vi "Pump Message Loop.vi"(7 "Manual Pump Select":enum32{"In", "Out"}(radio), 8 "error in (no error)":errorcluster) -> (0 "error out":errorcluster)   [LabVIEW 2020, in "Pump.lvlib"]
doc: "Message loop for handling messages pertaining to the acquisition of data from the hardware."
uses:
  Pump.lvlib
  support/PCT FGV CMD.ctl
  Acquisition State.ctl
  Pump Hardware Configuration.ctl
  support/Message Queue/Message Cluster.ctl
  support/Message Queue/Enqueue Message (Single).vi
  <vilib>/Utility/error.llb/Error Cluster From Error Code.vi
  <vilib>/ErrorRing/Error Ring.xnode
  support/Message Queue/Message Queue.lvlib
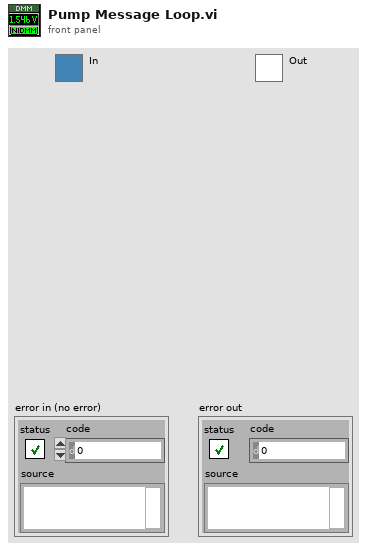
[diagram p1: front panel]
types:
  T1 = typedef "PCT FGV CMD.ctl" = enum16{"INIT", "GET", "SET"}
  T2 = typedef "PCT Data REFs.ctl" = cluster{"PLC AI Notifier":refnum<notifier>, "PS Data Queue":refnum<queue>, "BTN Queue":refnum<queue>, "PLC DI notifier":refnum<notifier>, "Timer notifier":refnum<notifier>, "DMM PS":refnum<notifier>, "DMM Gages":refnum<notifier>, "XYZ notifier":refnum<notifier>, "Test Notifier":refnum<notifier>, "Scanner notifier":refnum<notifier>, "OPC Notifier":refnum<notifier>, "HIDEN queue":refnum<queue>}
  T3 = typedef "Message Queue.lvlib/All Message Queues.ctl" = cluster{"UI":refnum<queue>, "Logging":refnum<queue>, "LOG":refnum<queue>, "ALARM":refnum<queue>, "Test":refnum<queue>, "Answer":refnum<queue>, "PLC":refnum<queue>, "DB":refnum<queue>, "Report":refnum<queue>, "OPC":refnum<queue>, "Procedure":refnum<queue>, "PalmSens":refnum<queue>, "SYS 7000 Reader":refnum<queue>, "SWITCH":refnum<queue>, "MOTOR":refnum<queue>, "MOTION":refnum<queue>, "HIDEN":refnum<queue>, "VALVE":refnum<queue>, "MFC":refnum<queue>, "PUMP IN":refnum<queue>, "PUMP OUT":refnum<queue>}
  T4 = typedef "Pump.lvlib/Pump Hardware Configuration.ctl" = cluster{"Pump  name":refnum<visa-resource-name>[], "Writer Queue":refnum<queue>, "Pump Info":cluster{"Pump Type":string, "Speed":i32, "Direction":u16, "Running":bool}, "Current Pump Name":refnum<visa-resource-name>, "Wait":dbl, "Next Step":string, "Reset":bool}
  T5 = cluster{"Type CMD":string, "Mode CMD":string, "Main CMD":string}
  T6 = typedef "Pump.lvlib/Acquisition State.ctl" = enum16{"Idle", "Initialized"}
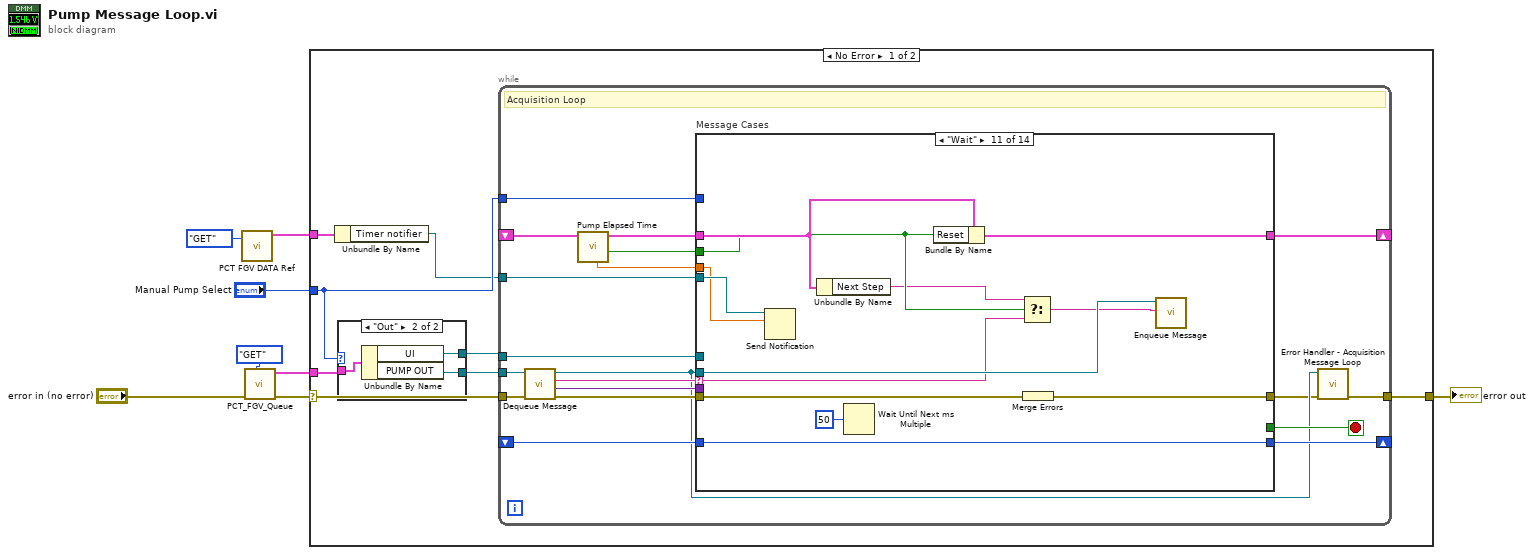
[diagram p0: block diagram]
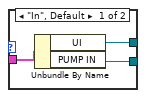
[diagram p2: hidden frame]
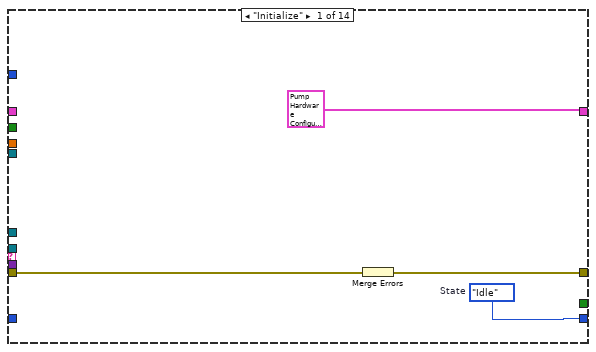
[diagram p3: hidden frame]
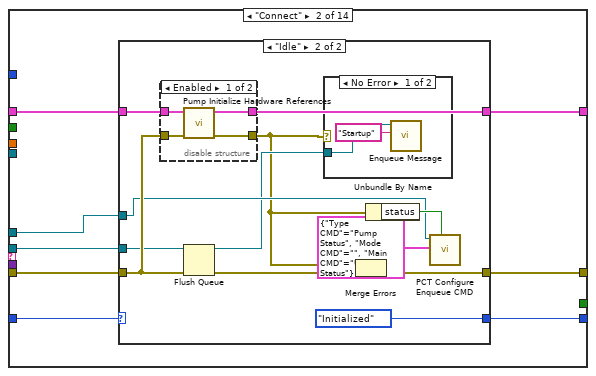
[diagram p4: hidden frame]
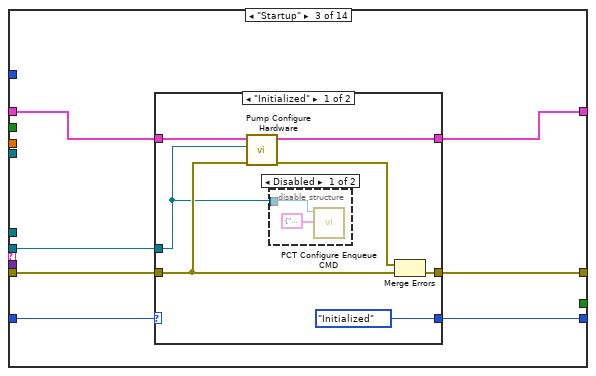
[diagram p8: hidden frame]
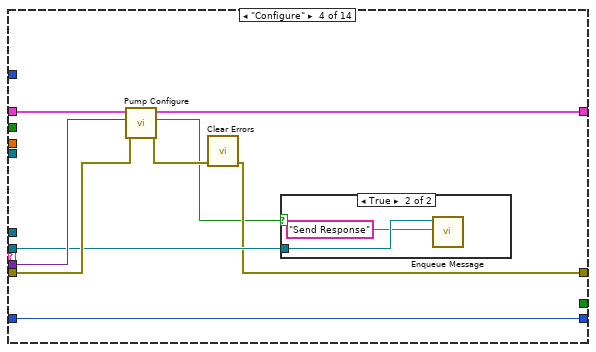
[diagram p11: hidden frame]
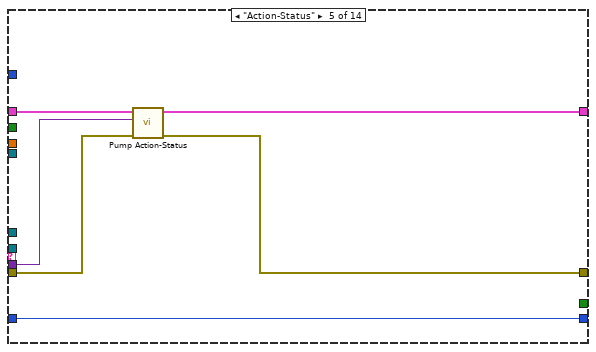
[diagram p13: hidden frame]
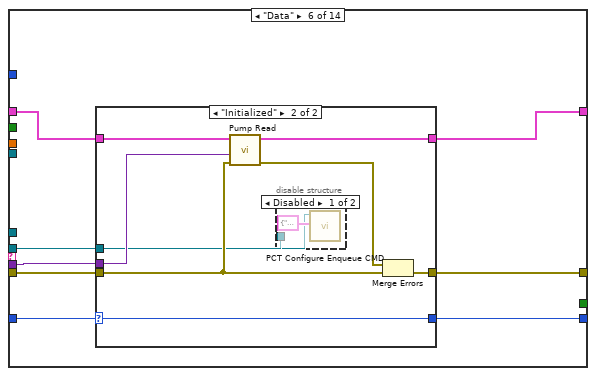
[diagram p14: hidden frame]
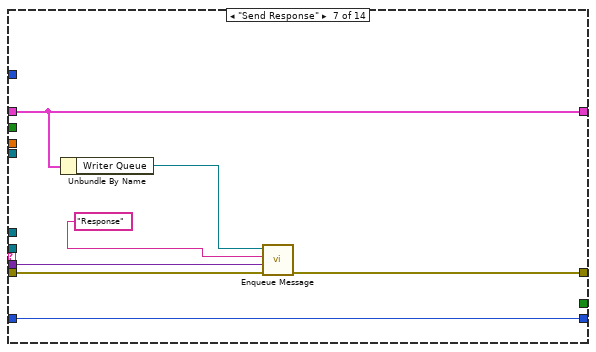
[diagram p17: hidden frame]
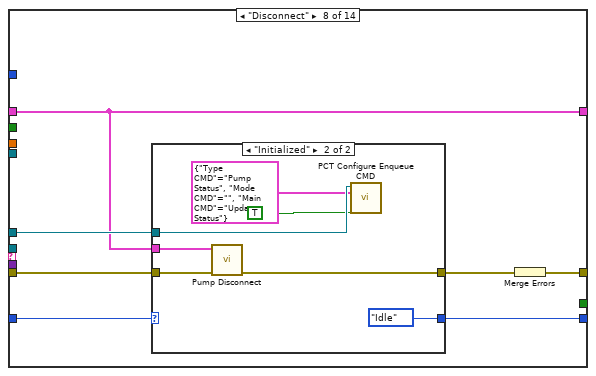
[diagram p18: hidden frame]
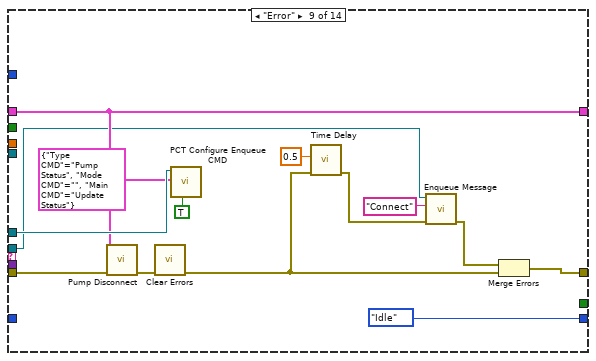
[diagram p20: hidden frame]
diagram:
  n1 = call "PCT FGV DATA Ref.vi"("CMD"=PCT_FGV_CMD."GET") -> ("Data REF"=w3:T2)  [unwired: 9 in, 1 out]
  n2 = call "PCT_FGV_Queue.vi"("CMD"=PCT_FGV_CMD."GET", "error in (no error)"="error in (no error)") -> ("error out"=w6:errorcluster, "Message Queues out"=w5:T3)  [unwired: 8 in]
  n3 = case shown="No Error" w6 {
    selector: w6 -> [w15 w220]
    tunnel: w5 -> [w11 _]
    tunnel: [w16 w220] -> w7
    tunnel: w3 -> [w14 _]
    tunnel: "Manual Pump Select" -> [w12 _]
    frame No Error {
      n4 = Unbundle By Name(w14) -> ("Timer notifier"=w9:refnum<notifier>)
      n5 = case shown="\"Out\"" w12 {
        tunnel: w11 -> [w19 w22]
        tunnel: [w18 w21] -> w13
        tunnel: [w17 w20] -> w10
        frame "In", Default {
          n6 = Unbundle By Name(w19) -> ("UI"=w17:refnum<queue>, "PUMP IN"=w18:refnum<queue>)
        }
        frame "Out" {
          n7 = Unbundle By Name(w22) -> ("UI"=w20:refnum<queue>, "PUMP OUT"=w21:refnum<queue>)
        }
      }
      n8 = while {
        tunnel: w13 -> [w36]
        shift-right: [w41] -> _
        shift-left: _ -> [w27]
        tunnel: w10 -> [w32]
        shift-right: [w34] -> _
        shift-left: _ -> [w35]
        tunnel: w15 -> [w39]
        tunnel: [w29] -> w16
        tunnel: w12 -> [w28]
        tunnel: w9 -> [w24]
        stop <- w40 stop-if-true
        # "Acquisition Loop"
        n9 = call "Dequeue Message.vi"("error in (no error)"=w39, "Message Queue"=w36) -> ("error out"=w38:errorcluster, "Message Data"=w37:variant, "Message"=w33:string, "dup Message Queue"=w31:refnum<queue>)  [unwired: 6 in]
        n10 = call "Pump Elapsed Time.vi"("Pump Refs in"=w27) -> ("Time has Elapsed"=w25:bool, "Pump Refs in"=w26:T4, "Elapsed Time (s)"=w23:dbl)  [unwired: 8 in]
        n11 = case "Message Cases" shown="\"Wait\"" w33 {
          selector: w33 -> [_ _ _ _ _ _ _ _ _ _ w175 _ _ w209]
          tunnel: w31 -> [_ w50 w78 w96 _ w117 _ _ w156 _ w178 _ w200 _]
          tunnel: w38 -> [w44 w51 w79 w99 w106 w116 w136 w144 w167 w172 w185 w196 w199 _]
          tunnel: [w45 w53 w81 w95 w105 w118 w135 w145 w168 w170 w184 w197 w205 w210] -> w30
          tunnel: w26 -> [_ w52 w80 w100 w107 w114 w133 w139 w163 w171 w182 w192 w204 w212]
          tunnel: [T4 {"Pump  name"=[], "Writer Queue"=refnum, "Pump Info"={"Pump Type"="", "Speed"=0, "Direction"=0, "Running"=FALSE}, "Current Pump Name"="", "Wait"=0.0, "Next Step"="", "Reset"=FALSE} ("Hardware Resources in") w49 w77 w97 w108 w115 w133 w139 w163 w171 w181 w187 w204 w212] -> w41
          tunnel: [_ _ _ _ _ _ _ _ _ _ _ _ TRUE _] -> w40
          tunnel: w37 -> [_ _ _ w101 w109 w111 w134 _ _ _ _ w194 w198 _]
          tunnel: w32 -> [_ w46 _ _ _ _ _ w140 w164 _ _ _ _ _]
          tunnel: w35 -> [_ w47 w75 w102 w110 w112 w137 w142 _ w169 w183 w195 w203 w211]
          tunnel: [w43 w48 w76 w102 w110 w113 w137 w141 Acquisition_State."Idle" ("State") w169 w183 w195 w203 w211] -> w34
          tunnel: w28 -> [_ _ _ _ _ _ _ _ _ _ _ w188 _ _]
          tunnel: w25 -> [_ _ _ _ _ _ _ _ _ _ w177 _ _ _]
          tunnel: w24 -> [_ _ _ _ _ _ _ _ _ _ w180 _ _ _]
          tunnel: w23 -> [_ _ _ _ _ _ _ _ _ _ w173 _ _ _]
          frame "Initialize" {
            w43 = Acquisition_State."Idle"  # State
            # "Initialize  - Initialize is currently a no-op.  The hardware initialization takes place in the 'Start' message."
            n12 = Merge Errors(w44) -> (w45:errorcluster)
          }
          frame "Connect" {
            # "Start - Configure and start the acquisition."
            n13 = case shown="\"Idle\"" w47 {
              selector: w47 -> [w54 _]
              tunnel: [w55 w67] -> w53
              tunnel: w52 -> [w56 w66]
              tunnel: w51 -> [w55 w64]
              tunnel: w50 -> [_ w63]
              tunnel: [w56 w62] -> w49
              tunnel: [w54 Acquisition_State."Initialized" ("Acquisition State")] -> w48
              tunnel: w46 -> [_ w59]
              frame "Initialized" {
                # "The system is already acquiring. Ignore the \"Start\" message."
              }
              frame "Idle" {
                # "If the system is idle, start the acquisition."
                n14 = disable-structure shown="Enabled" {
                  disable-tunnel: w66 -> [w73 w74]
                  disable-tunnel: w64 -> [w72 _]
                  disable-tunnel: [w71 w74] -> w62
                  disable-tunnel: [w70 _] -> w57
                  frame Enabled {
                    n15 = call "Pump Initialize Hardware References.vi"("error in (no error)"=w72, "Hardware Resources in"=w73) -> ("error out"=w70:errorcluster, "Hardware Resources out"=w71:T4)  [unwired: 8 in]
                  }
                  frame Disabled {
                  }
                }
                n16 = Flush Queue(queue=w63) -> (queue out=w58:refnum<queue>)  [unwired: 1 in, 2 out]
                n17 = case shown="No Error" w57 {
                  tunnel: w58 -> [w69 _]
                  frame No Error {
                    n18 = call-poly "Enqueue Message.vi"("Message"="Startup", "Message Queue"=w69) -> ()  [unwired: 8 in, 2 out]
                  }
                  frame Error {
                  }
                }
                n19 = Merge Errors(w57, w64) -> (w67:errorcluster)
                n20 = Unbundle By Name(w57) -> ("status"=w60:bool)
                n21 = call "PCT Configure Enqueue CMD.vi"("Parameter Data"=w60, "CMD"=T5 {"Type CMD"="Pump Status", "Mode CMD"="", "Main CMD"="Update Status"}, "CMD Queue in"=w59) -> ()  [unwired: 6 in, 3 out]
              }
            }
          }
          frame "Startup" {
            # "Start - Configure and start the acquisition."
            n22 = case shown="\"Initialized\"" w75 {
              selector: w75 -> [_ w91]
              tunnel: [w88 w92] -> w81
              tunnel: w80 -> [w87 w93]
              tunnel: w79 -> [w84 w92]
              tunnel: w78 -> [w82 _]
              tunnel: [w86 w93] -> w77
              tunnel: [Acquisition_State."Initialized" ("Acquisition State") w91] -> w76
              frame "Initialized" {
                # "If the system is idle, start the acquisition."
                n23 = call "Pump Configure Hardware.vi"("error in (no error)"=w84, "DMM"=w82, "Hardware Resources in"=w87) -> ("error out"=w83:errorcluster, "Hardware Resources out"=w86:T4)  [unwired: 7 in]
                n24 = disable-structure shown="Disabled" {
                  disable-tunnel: w82 -> [w89 _]
                  frame Disabled {
                    n25 = call "PCT Configure Enqueue CMD.vi"("CMD"=T5 {"Type CMD"="Single", "Mode CMD"="Single", "Main CMD"="Data"}, "CMD Queue in"=w89) -> ()  [unwired: 7 in, 3 out]
                  }
                  frame Enabled {
                  }
                }
                n26 = Merge Errors(w83, w84) -> (w88:errorcluster)
              }
              frame "Idle" {
                # "The system is already acquiring. Ignore the \"Start\" message."
              }
            }
          }
          frame "Configure" {
            # "Start - Configure and start the acquisition."
            n27 = call "Pump Configure.vi"("error in (no error)"=w99, "Message Data"=w101, "Data Cluster"=w100) -> ("error out"=w98:errorcluster, "Send Resp"=w94:bool, "Data Cluster out"=w97:T4)  [unwired: 6 in]
            n28 = call <vilib>:"Clear Errors.vi"("error in (no error)"=w98) -> ("error out"=w95:errorcluster)  [unwired: 5 in, 1 out]
            n29 = case shown="True" w94 {
              tunnel: w96 -> [_ w104]
              frame False {
              }
              frame True {
                n30 = call-poly "Enqueue Message.vi"("Message"="Send Response", "Message Queue"=w104) -> ()  [unwired: 8 in, 2 out]
              }
            }
          }
          frame "Action-Status" {
            # "Start - Configure and start the acquisition."
            n31 = call "Pump Action-Status.vi"("error in (no error)"=w106, "Message Data"=w109, "Data Cluster"=w107) -> ("error out"=w105:errorcluster, "Data Cluster out"=w108:T4)  [unwired: 7 in]
          }
          frame "Data" {
            # "Acquire - Acquire data from the hardware. Since this is a continuous acquisition, this message will always message itself to run again."
            n32 = case shown="\"Initialized\"" w112 {
              selector: w112 -> [w119 w125]
              tunnel: [w120 w129] -> w118
              tunnel: w117 -> [_ w122]
              tunnel: w116 -> [w120 w123]
              tunnel: [w121 w127] -> w115
              tunnel: w114 -> [w121 w126]
              tunnel: [w119 w125] -> w113
              tunnel: w111 -> [_ w124]
              frame "Idle" {
              }
              frame "Initialized" {
                # "Read  data"
                n33 = call "Pump Read.vi"("error in (no error)"=w123, "Message Data"=w124, "Hardware Resources in"=w126) -> ("error out"=w128:errorcluster, "Hardware Resources out"=w127:T4)  [unwired: 5 in, 2 out]
                n34 = disable-structure shown="Disabled" {
                  disable-tunnel: w122 -> [w130 _]
                  frame Disabled {
                    n35 = call "PCT Configure Enqueue CMD.vi"("CMD"=T5 {"Type CMD"="Single", "Mode CMD"="Single", "Main CMD"="Data"}, "CMD Queue in"=w130) -> ()  [unwired: 7 in, 3 out]
                  }
                  frame Enabled {
                  }
                }
                n36 = Merge Errors(w128, w123) -> (w129:errorcluster)
              }
            }
          }
          frame "Send Response" {
            # "Acquire - Acquire data from the hardware. Since this is a continuous acquisition, this message will always message itself to run again."
            n37 = Unbundle By Name(w133) -> ("Writer Queue"=w132:refnum<queue>)
            n38 = call-poly "Enqueue Message.vi"("error in (no error)"=w136, "Message Data"=w134, "Message"="Response", "Message Queue"=w132) -> ("error out"=w135:errorcluster)  [unwired: 6 in, 1 out]
          }
          frame "Disconnect" {
            # "Stop - Stop the Acquisition."
            n39 = case shown="\"Initialized\"" w142 {
              selector: w142 -> [w146 _]
              tunnel: w144 -> [w147 w154]
              tunnel: [w147 w153] -> w143
              tunnel: w139 -> [_ w151]
              tunnel: [w146 Acquisition_State."Idle" ("State")] -> w141
              tunnel: w140 -> [_ w150]
              frame "Idle" {
                # "The system is already idle. Ignore the \"Stop\" message."
              }
              frame "Initialized" {
                # "If the system is acquiring, stop the acquisition."
                n40 = call "Pump Disconnect.vi"("error in (no error)"=w154, "Hardware Resources in"=w151) -> ("error out"=w153:errorcluster)  [unwired: 9 in]
                n41 = call "PCT Configure Enqueue CMD.vi"("Parameter Data"=TRUE, "CMD"=T5 {"Type CMD"="Pump Status", "Mode CMD"="", "Main CMD"="Update Status"}, "CMD Queue in"=w150) -> ()  [unwired: 6 in, 3 out]
              }
            }
            n42 = Merge Errors(w143) -> (w145:errorcluster)
          }
          frame "Error" {
            # "Stop - Stop the Acquisition."
            n43 = call "Pump Disconnect.vi"("error in (no error)"=w167, "Hardware Resources in"=w163) -> ("error out"=w166:errorcluster)  [unwired: 9 in]
            n44 = call <vilib>:"Clear Errors.vi"("error in (no error)"=w166) -> ("error out"=w159:errorcluster)  [unwired: 5 in, 1 out]
            n45 = call "PCT Configure Enqueue CMD.vi"("Parameter Data"=TRUE, "CMD"=T5 {"Type CMD"="Pump Status", "Mode CMD"="", "Main CMD"="Update Status"}, "CMD Queue in"=w164) -> ()  [unwired: 6 in, 3 out]
            n46 = call "Time Delay"("error in (no error)"=w159, "Delay Time (s)"=0.5) -> ("error out"=w158:errorcluster)  [unwired: 9 in]
            n47 = call-poly "Enqueue Message.vi"("error in (no error)"=w158, "Message"="Connect", "Message Queue"=w156) -> ("error out"=w157:errorcluster)  [unwired: 7 in, 1 out]
            n48 = Merge Errors(w157, w159) -> (w168:errorcluster)
          }
          frame "---Copy This Frame---" {
            # "Duplicate this frame when creating new messages.  Change this comment in the duplicated frame to describe this message."
            n49 = Merge Errors(w172) -> (w170:errorcluster)
          }
          frame "Wait" {
            # "Duplicate this frame when creating new messages.  Change this comment in the duplicated frame to describe this message."
            n50 = Send Notification(notification=w173, notifier=w180) -> ()  [unwired: 1 in, 2 out]
            n51 = Unbundle By Name(w182) -> ("Next Step"=w176:string)
            n52 = Wait Until Next ms Multiple(millisecond multiple=u32 50) -> ()  [unwired: 1 out]
            n53 = Bundle By Name(cluster=w182, "Reset"=w177) -> (w181:T4)
            n54 = Select(t=w176, s=w177, f=w175) -> (s? t:f=w174:string)
            n55 = Merge Errors(w185) -> (w184:errorcluster)
            n56 = call-poly "Enqueue Message.vi"("Message"=w174, "Message Queue"=w178) -> ()  [unwired: 8 in, 2 out]
          }
          frame "Update Settings" {
            # "New settings are available, update the current ones stored in the shift register with the settings sent as part of the message"
            n57 = Variant To Data(type=w192, Variant=w194) -> (data=w191:T4, error out=w193:errorcluster)  [unwired: 1 in]
            n58 = Select(t=w192, s=w193, f=w191) -> (s? t:f=w190:T4)
            n59 = Unbundle By Name(w190) -> ("Pump  name"=w189:refnum<visa-resource-name>[])
            n60 = Merge Errors(w196) -> (w197:errorcluster)
            n61 = Index Array(array=w189, index=w188) -> (element=w186:refnum<visa-resource-name>)
            n62 = Bundle By Name(cluster=w190, "Current Pump Name"=w186) -> (w187:T4)
          }
          frame "Exit" {
            # "Release the EXA queue reference"
            # "Stop the VI"
            # "Exit - Send the Exit message to the UI Message Handler."
            n63 = Variant To Data(type=TRUE, Variant=w198) -> (data=w202:bool)  [unwired: 1 in, 1 out]
            n64 = case shown="True" w202 {
              tunnel: w200 -> [_ w208]
              frame False {
              }
              frame True {
                n65 = call-poly "Enqueue Message.vi"("Message"="Exit", "Message Queue"=w208) -> ()  [unwired: 8 in, 2 out]
              }
            }
            n66 = Merge Errors(w199) -> (w205:errorcluster)
          }
          frame Default {
            # "'Default' case only runs if there is a message that isn't defined in any of the other cases.  Output a programming error."
            n67 = xnode "Error Ring"("parameter 0"=w209) -> ("error out"=w210:errorcluster)
          }
        }
        n68 = call "Error Handler - Acquisition Message Loop.vi"("error in (no error)"=w30, "Message Queue"=w31) -> ("dup error in"=w29:errorcluster)  [unwired: 8 in, 1 out]
      }
    }
    frame Error {
    }
  }
  "error out" <- w7
